vi "Destroy.vi"   [LabVIEW 2021, in "Field_RnD_Services_LIBSSH2_Toolkit.lvlib" / "Channel.lvclass"]
doc: "Deallocates, or frees, the memory allocated for the libssh2lv shared library Channel struct represented by this Channel object. After this is called, the object can no longer be used in the application without causing a segmentation fault, i.e. crashing LabVIEW. This VI must be called to avoid leaking memory or running Out-of-Memory (OOM) on resource-constrained systems."
uses:
  220524-VNA RP FLAT.llb/Channel.lvclass
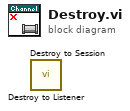
[diagram p0: block diagram]
diagram:
  n1 = call "Destroy to Listener.vi"() -> ()  [unwired: 10 in, 2 out]
  n2 = call "Destroy to Session.vi"() -> ()  [unwired: 10 in, 2 out]
